vi "Generate Process.vi"(8 "error in (no error)":errorcluster, 11 "Process Generator In":refnum<class "Process Generator.lvclass">) -> (0 "error out":errorcluster, 3 "Process Generator Out":refnum<class "Process Generator.lvclass">)   [LabVIEW 2020, in "Process Generation.lvlib" / "Process Generator.lvclass"]
uses:
  Process Generator.lvclass
  Process Generator.lvclass/Process Generator.ctl
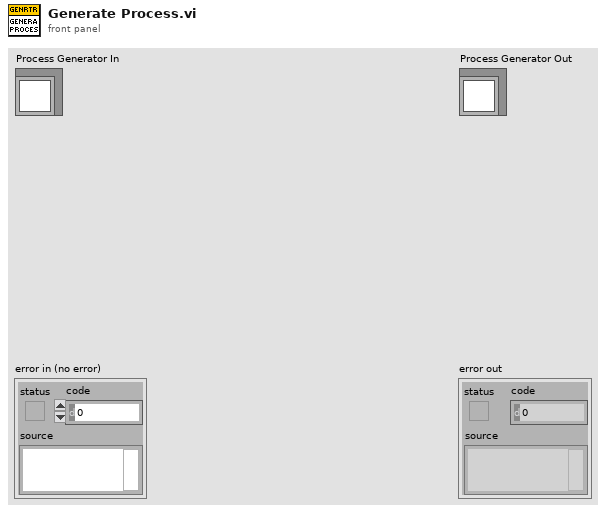
[diagram p1: front panel]
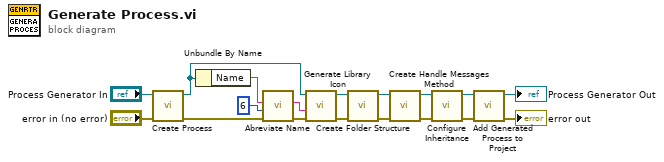
[diagram p0: block diagram]
diagram:
  n1 = call "Create Process.vi"("error in (no error)"="error in (no error)", "Process Generator in"="Process Generator In") -> ("error out"=w4:errorcluster, "Process Generator out"=w8:refnum<class "Process Generator.lvclass">)  [unwired: 8 in]
  n2 = Unbundle By Name(w8) -> ("Name"=w7:string)
  n3 = call "Abreviate Name.vi"("error in (no error)"=w4, "Max Length"=6, "Long Name"=w7) -> ("error out"=w6:errorcluster, "Abreviated Name"=w1:string)  [unwired: 7 in]
  n4 = call "Generate Library Icon.vi"("error in (no error)"=w6, "Overlay Text"=w1, "Process Generator In"=w8) -> ("error out"=w5:errorcluster, "Process Generator Out"=w3:refnum<class "Process Generator.lvclass">)  [unwired: 6 in, 1 out]
  n5 = call "Create Folder Structure.vi"("error in (no error)"=w5, "Process Generator In"=w3) -> ("error out"=w10:errorcluster, "Process Generator Out"=w2:refnum<class "Process Generator.lvclass">)  [unwired: 8 in]
  n6 = call "Create Handle Messages Method.vi"("error in (no error)"=w10, "Process Generator in"=w2) -> ("error out"=w9:errorcluster, "Process Generator out"=w11:refnum<class "Process Generator.lvclass">)  [unwired: 8 in]
  n7 = call "Configure Inheritance.vi"("error in (no error)"=w9, "Process Generator in"=w11) -> ("error out"=w18:errorcluster, "Process Generator out"=w12:refnum<class "Process Generator.lvclass">)  [unwired: 8 in]
  n8 = call "Add Generated Process to Project.vi"("error in (no error)"=w18, "Process Generator in"=w12) -> ("error out"=→"error out":errorcluster, "Process Generator out"=→"Process Generator Out":refnum<class "Process Generator.lvclass">)  [unwired: 8 in]
